vi "DecodeBoardCapability.vi"(11 "CapabilityWord":u16) -> (2 "NAVX_BOARD_YAW_AXIS":T1, 3 "NAVX_BOARD_CAPABILITY":T2)   [LabVIEW 2014, in "navX-MXP IMU.lvlib"]
uses:
  navX-MXP IMU.lvlib
  TypeDefs/Value TypeDefs/navX NAVX_BOARD_CAPABILITY.ctl
  TypeDefs/Value TypeDefs/navX NAVX_BOARD_YAW_AXIS.ctl
  TypeDefs/Value TypeDefs/navX NAVX_CAPABILITY_FLAGS.ctl
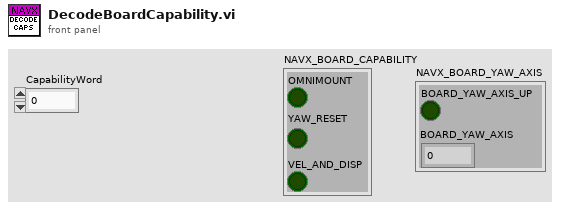
[diagram p1: front panel]
types:
  T1 = typedef "navX-MXP IMU.lvlib/navX NAVX_BOARD_YAW_AXIS.ctl" = cluster{"BOARD_YAW_AXIS_UP":bool, "BOARD_YAW_AXIS":u8}
  T2 = typedef "navX-MXP IMU.lvlib/navX NAVX_BOARD_CAPABILITY.ctl" = cluster{"OMNIMOUNT":bool, "YAW_RESET":bool, "VEL_AND_DISP":bool}
  T3 = typedef "navX-MXP IMU.lvlib/navX NAVX_CAPABILITY_FLAGS.ctl" = u8
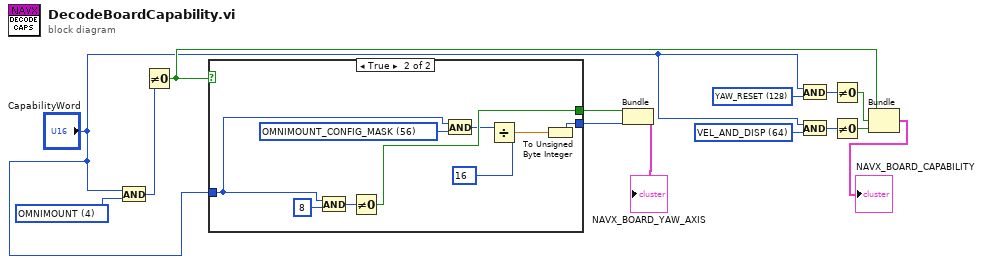
[diagram p0: block diagram]
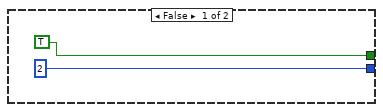
[diagram p2: hidden frame]
diagram:
  w6 = T3 64 items=["OMNIMOUNT"=4, "VEL_AND_DISP "=64, "YAW_RESET"=128, "OMNIMOUNT_CONFIG_MASK"=56] ("NAVX_CAPABILITY_FLAG")
  w10 = T3 128 items=["OMNIMOUNT"=4, "VEL_AND_DISP "=64, "YAW_RESET"=128, "OMNIMOUNT_CONFIG_MASK"=56] ("NAVX_CAPABILITY_FLAG")
  w11 = T3 4 items=["OMNIMOUNT"=4, "VEL_AND_DISP "=64, "YAW_RESET"=128, "OMNIMOUNT_CONFIG_MASK"=56] ("NAVX_CAPABILITY_FLAG")
  n1 = And(x="CapabilityWord", y=w11) -> (x .and. y?=w4:u16)
  n2 = Not Equal To 0?(x=w4) -> (x != 0?=w12:bool)
  n3 = case shown="True" w12 {
    tunnel: [TRUE w23] -> w14
    tunnel: [u8 2 w17] -> w13
    tunnel: "CapabilityWord" -> [_ w21]
    frame False {
    }
    frame True {
      w22 = T3 56 items=["OMNIMOUNT"=4, "VEL_AND_DISP "=64, "YAW_RESET"=128, "OMNIMOUNT_CONFIG_MASK"=56] ("NAVX_CAPABILITY_FLAG")
      n4 = And(x=w21, y=u8 8 ("Read Size")) -> (x .and. y?=w24:u16)
      n5 = Not Equal To 0?(x=w24) -> (x != 0?=w23:bool)
      n6 = And(x=w21, y=w22) -> (x .and. y?=w20:u16)
      n7 = Divide(x=w20, y=u8 16 ("Read Size")) -> (x/y=w18:dbl)
      n8 = To Unsigned Byte Integer(number=w18) -> (unsigned 8bit integer=w17:u8)
    }
  }
  n9 = Bundle(w14, w13) -> (→"NAVX_BOARD_YAW_AXIS":cluster{bool, u8})  [unwired: 1 in]
  n10 = And(x="CapabilityWord", y=w10) -> (x .and. y?=w9:u16)
  n11 = And(x="CapabilityWord", y=w6) -> (x .and. y?=w7:u16)
  n12 = Not Equal To 0?(x=w9) -> (x != 0?=w8:bool)
  n13 = Not Equal To 0?(x=w7) -> (x != 0?=w5:bool)
  n14 = Bundle(w12, w8, w5) -> (→"NAVX_BOARD_CAPABILITY":cluster{bool, bool, bool})  [unwired: 1 in]
